vi "MetaClientReadStop.vi"() -> (0 "ServerStop":bool)   [LabVIEW 2017]
panel:
  out "data out":string
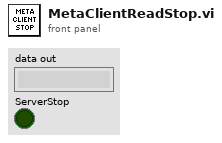
[diagram p1: front panel]
types:
  T1 = enum16{"Standard", "Buffered", "CRLF", "Immediate"}
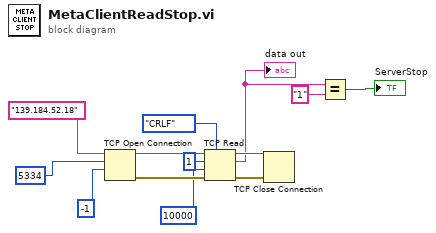
[diagram p0: block diagram]
diagram:
  n1 = TCP Open Connection(address="139.184.52.18", remote port or service name=u16 5334, timeout ms (60000)=-1) -> (connection ID=w13:refnum<k5>, error out=w12:errorcluster)  [unwired: 2 in]
  n2 = TCP Read(connection ID=w13, bytes to read=1, error in (no error)=w12, 7:T1."CRLF" ("mode (standard)"), 9:10000 ("timeout ms (25000)")) -> (connection ID out=w9:refnum<k5>, data out=w3:string, error out=w10:errorcluster)
  "data out" <- w3
  n3 = TCP Close Connection(connection ID=w9, error in (no error)=w10) -> ()  [unwired: 1 in, 2 out]
  n4 = Equal?(x=w3, y="1") -> (x = y?=→"ServerStop":bool)
